vi "ProdaNG.TestValueResult.Get.vi"(8 "error in (no error)":errorcluster, 9 "testValueId":i32, 10 "testStepResultId":string, 11 "dbHandle":i32) -> (0 "error out":errorcluster, 2 "TestValueResult":T1, 3 "dbHandle":i32)   [LabVIEW 2016]
doc: "This function changes the process step result, which is defined by a ProcessStepResult structure. A process step result can either be set intentionally or leave the check of the test step results and the resulting changes to the DLL. In case, that the DLL changes the Process Result, the mdTime of the according Product is set to the current time and the mdProcessStepId is set to this process step. \nThe automatic check stands to the following rule:\n1. It is checked, if all test steps have the Status IO.\nIf the result of the test is IO, the status 1 (IO) is set in the test value result, otherwise the status 0 (NIO), respective 5 (IO Repeat) or 6 (NIO Repeat) in case of a repeat.\nParameter:\nhandle is an Integer, which is returned by the function Login() at the creation of a new connection.\nisRepeat shows, if this step is a repeat.\nprocessStepResult is a pointer on a ProcessStepResult structure, which elements must be prefilled. The structure must be defined and filled in the calling program. Changes can only be made on the elements StatusId, startTime and endTime. If the Endtime is not set, it is automatically filled with the current time by the DLL. \nThe element statusId is of particular importance:\nIf this element is passed with the value -1, the DLL makes a check on the test step results and sets the changeable elements automatically. Otherwise the returned values for status, start time and end time are set.\n\nReturncodes:\n0 No error\n< 0 ORACLE Error code\n6 (ERROR_INVALID_HANDLE) in case of an invalid handle\n1403 Record does not exist"
uses:
  Controls/ProdaNG.TestValueResult.ctl
  Controls/ProdaNG.TestValueResultSize.ctl
  prodllNG.dll
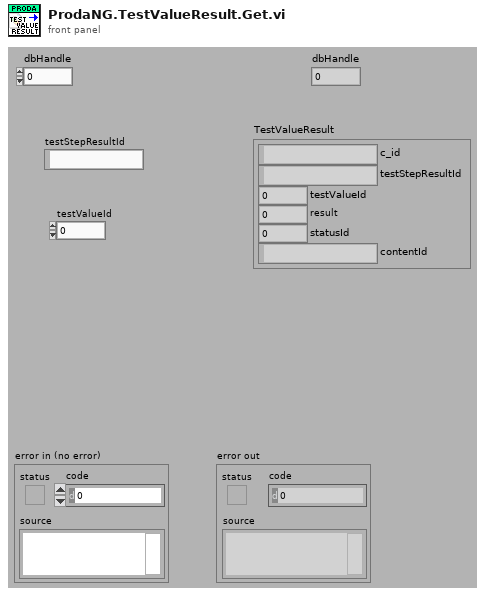
[diagram p1: front panel]
types:
  T1 = typedef "ProdaNG.TestValueResult.ctl" = cluster{"c_id":string, "testStepResultId":string, "testValueId":i32, "result":dbl, "statusId":i32, "contentId":string}
  T2 = typedef "ProdaNG.TestValueResultSize.ctl" = cluster{"c_id":i32, "testStepResultId":i32, "testValueId":i32, "result":i32, "statusId":i32, "contentId":i32}
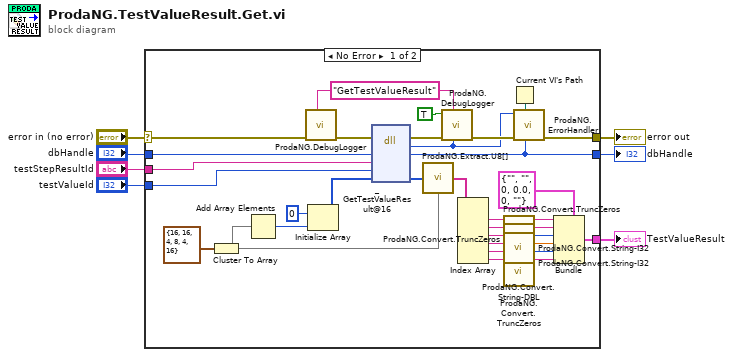
[diagram p0: block diagram]
diagram:
  n1 = case shown="No Error" "error in (no error)" {
    selector: "error in (no error)" -> [w34 w43]
    tunnel: [w32 w43] -> w6
    tunnel: [w31 w42] -> w5
    tunnel: "dbHandle" -> [w33 w42]
    tunnel: [w10 _] -> w3
    tunnel: "testStepResultId" -> [w9 _]
    tunnel: "testValueId" -> [w8 _]
    frame No Error {
      w40 = "GetTestValueResult" ("cmd")
      n2 = Cluster To Array(cluster=T2 {"c_id"=16, "testStepResultId"=16, "testValueId"=4, "result"=8, "statusId"=4, "contentId"=16} ("TestValueResultSize")) -> (array=w28:i32[])
      n3 = Add Array Elements(numeric array=w28) -> (sum=w29:i32)
      n4 = call "ProdaNG.DebugLogger.vi"("cmd"=w40, "error in (no error)"=w34) -> ("error out"=w35:errorcluster)  [unwired: 9 in]
      n5 = Initialize Array(u8 0 ("element"), w29) -> (w11:u8[])
      n6 = dll-call lib="D:/Maszup/WABCO/SVN/LineTraceSystem/SOFTWARE/sources/Database/ProdaNG/prodllNG.dll" fn="_GetTestValueResult@16" ("ProDll.dll:InitProDll")(error in=w35, "dbHandle"=w33, "testStepResultId"=w9, "testValueId"=w8, "testValueResult"=w11) -> (error out=w38:errorcluster, "return type"=w36:i32, "dbHandle"=w31:i32, "testValueResult"=w12:u8[])  [unwired: 4 in, 1 out]
      n7 = call "ProdaNG.Extract.U8[].vi"("unsigned byte array"=w12, "Sizes"=w28) -> ("Elements"=w13:string[])
      n8 = call "ProdaNG.DebugLogger.vi"("return type"=w36, "cmd"=w40, "error in (no error)"=w38, "done? (F)"=TRUE) -> ("error out"=w37:errorcluster)  [unwired: 7 in]
      n9 = Index Array(array=w13) -> (element #1=w20:string, element #2=w19:string, element #3=w27:string, element #4=w24:string, element #5=w16:string, element #6=w23:string)  [unwired: 6 in]
      n10 = call "ProdaNG.Convert.TruncZeros.vi"("string with \\0s"=w20) -> ("LV string"=w22:string)  [unwired: 10 in]
      n11 = call "ProdaNG.Convert.TruncZeros.vi"("string with \\0s"=w19) -> ("LV string"=w21:string)  [unwired: 10 in]
      n12 = call "ProdaNG.Convert.String-I32.vi"("unsigned byte string"=w27) -> ("32bit integer"=w26:i32)  [unwired: 10 in]
      n13 = call "ProdaNG.Convert.String-DBL.vi"("unsigned byte string"=w24) -> ("dbl integer"=w25:dbl)  [unwired: 10 in]
      n14 = call "ProdaNG.Convert.String-I32.vi"("unsigned byte string"=w16) -> ("32bit integer"=w15:i32)  [unwired: 10 in]
      n15 = call "ProdaNG.Convert.TruncZeros.vi"("string with \\0s"=w23) -> ("LV string"=w17:string)  [unwired: 10 in]
      n16 = Current VI's Path() -> (path=w41:path)
      n17 = call "ProdaNG.ErrorHandler.vi"("dbHandleIn"=w31, "Path"=w41, "error in"=w37, "output_parameter"=w36) -> ("error out"=w32:errorcluster)  [unwired: 7 in]
      n18 = Bundle(cluster=T1 {"c_id"="", "testStepResultId"="", "testValueId"=0, "result"=0.0, "statusId"=0, "contentId"=""} ("TestValueResult"), "c_id"=w22, "testStepResultId"=w21, "testValueId"=w26, "result"=w25, "statusId"=w15, "contentId"=w17) -> (w10:T1)
    }
    frame Error {
    }
  }
  "error out" <- w6
  "dbHandle" <- w5
  "TestValueResult" <- w3
